vi "Set Force.vi"(0 "class data in":refnum<class "MB_ENGINE.lvclass">, 5 "percent":u16, 11 "error in (no error)":errorcluster) -> (4 "class data out":refnum<class "MB_ENGINE.lvclass">, 15 "error out":errorcluster)   [LabVIEW 2019, in "MB_ENGINE.lvclass"]
uses:
  MB_ENGINE.lvclass
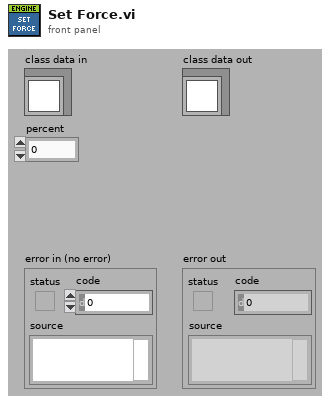
[diagram p1: front panel]
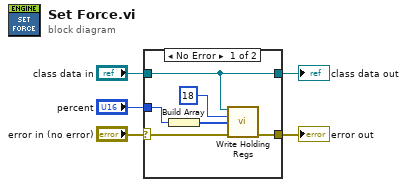
[diagram p0: block diagram]
diagram:
  n1 = case shown="No Error" "error in (no error)" {
    selector: "error in (no error)" -> [w9 w13]
    tunnel: [w8 w13] -> w4
    tunnel: "class data in" -> [w11 w12]
    tunnel: [w11 w12] -> w2
    tunnel: "percent" -> [w7 _]
    frame No Error {
      n2 = Build Array(w7) -> (w6:u16[])
      n3 = call-dynamic "Write Holding Regs.vi"("reference in"=w11, "starting address"=u16 18, "Regs"=w6, "error in (no error)"=w9) -> ("error out"=w8:errorcluster)  [unwired: 11 in]
    }
    frame Error {
    }
  }
  "error out" <- w4
  "class data out" <- w2
